vi "Lab6_DPSK2.vi"() -> ()   [LabVIEW 2019]
uses:
  <vilib>/addons/Modulation/Analog/support/mod_Set Error Source.vi
  <vilib>/addons/Modulation/Digital/Support/Common/Validators/mod_AWGN Validate.vi
  <vilib>/addons/Modulation/Digital/Impairments/subVIs/mod_createSeeds.vi
  <vilib>/addons/Modulation/Digital/Support/Common/Validators/mod_Validate Samples Per Symbol.vi
  <vilib>/addons/Modulation/Analog/support/Validators/mod_Validate Complex Waveform.vi
  <vilib>/addons/Modulation/Analog/support/Validators/mod_WFErrorHandler.vi
  <vilib>/addons/Modulation/Digital/Support/Common/Validators/mod_Generate Filter Coefficients Validate.vi
  <vilib>/addons/Modulation/Digital/General/subVIs/mod_Generate Filter Coefficients.vi
  <vilib>/addons/Modulation/Digital/General/MT Generate PSK System Parameters(M).vi
  <vilib>/addons/Modulation/Digital/General/MT Generate PSK Synchronization Parameters (bit array).vi
  <vilib>/addons/Modulation/Digital/General/subVIs/mod_Generate Bits PN Sequence.vi
  <vilib>/Analysis/1siggen.llb/Gaussian White Noise (obs 90).vi
  <vilib>/addons/Modulation/Analog/MT Upconvert Baseband (Real).vi
  <vilib>/addons/Modulation/Digital/Demodulation/MT Calculate BER After Trigger (PN Sequence).vi
  <vilib>/addons/Modulation/Digital/General/MT Format Eye Diagram (complex).vi
  <vilib>/express/express analysis/Spectral/Block/exnSpectralBlock spectral measurements RMS poly.vi
  <vilib>/express/express analysis/Spectral/Block/exnSpectralBlock spectral measurements RMS WFM.vi
  <vilib>/express/express analysis/Spectral/XNode/ExpressSpectralMeasurementsBlockNode.xnode
  <vilib>/addons/Modulation/niDMT.lvlib
  <vilib>/addons/Modulation/niAMT.lvlib
panel:
  in  "Tab Control 2":T1(tab)
  out "bassband wfm1":cluster{"t0":dbl, "dt":dbl, "Y":dbl[]}(graph)
  out "bassband wfm2":cluster{"t0":dbl, "dt":dbl, "Y":dbl[]}(graph)
  out "passband wfm":waveform(dbl)(graph)
  out "Spectral":cluster{"f0":dbl, "df":dbl, "magnitude":dbl[]}(graph)
  in  "Tab Control":enum32{" Constellation", "Eye Diagram"}(tab)
  out "Constellation":T2(graph)
  out "Eye Diagram":cluster{"t0":dbl, "dt":dbl, "Y":dbl[]}[](graph)
  in  "carrier frequency (Hz)":dbl min=-0.5 max=0.5 format="%.0p"
  in  "PSK type":u16(ring) items=["normal", "shifted", "offset"]
  out "Transmitted bitstream":i8[](array[numeric])
  out "Receive bit stream":i8[](array[numeric])
  in  "Eb/N0 (10 dB)":dbl(knob)=10.0 scale=0.0..60.0
  in  "symbol rate (Hz)":dbl=1.0 format="%.0p"
  in  "M-PSK(4)":i32(ring) items=["2"=2, "4"=4, "8"=8, "16"=16]
  in  "stop":bool
  in  "pulse shaping filter":u16(ring) items=["none", "Raised Cosine", "Root Raised Cos", "Gaussian"]
  # "DPSK and Offset-PSK"
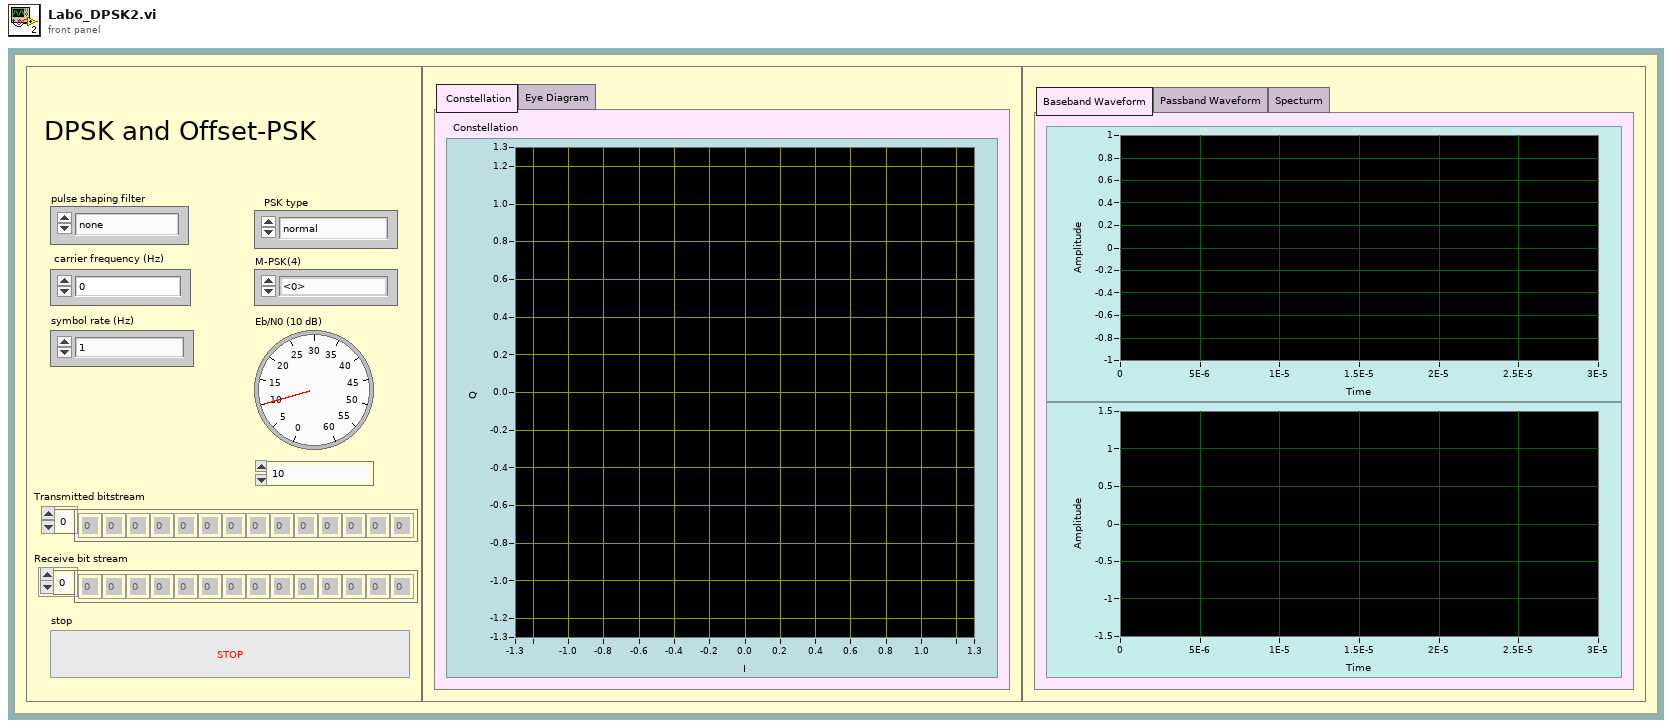
[diagram p1: front panel]
types:
  T1 = enum32{"Baseband Waveform", "Passband Waveform", "Specturm"}
  T2 = cluster{"Decimated Array":dbl[], "Decimated Array":dbl[]}[]
  T3 = enum16{"FSK", "PSK", "QAM", "MSK", "PAM", "ASK", "CPM"}
  T4 = cluster{"averaging mode":u16, "weighting mode":u16, "number of averages":u32}
  T5 = cluster{"dB On (F)":bool, "unwrap phase (F)":bool, "convert to degree (F)":bool}
  T6 = cluster{"samples per symbol (16)":i32, "symbol map":cdb[], "differential PSK":enum16{"disable", "enable"}, "PSK type":u16}
  T7 = cluster{"expected sync location (symbols)":i32, "sync sequence":cdb[], "sync location uncertainty (symbols)":i32, "sync indent (symbols)":i32}
  T8 = typedef "niAMT.lvlib/Complex Data Waveform.ctl" = cluster{"t0":dbl, "dt":dbl, "Y":cdb[]}
  T9 = cluster{"constellation":dbl[], "oversampled data":dbl[]}[]
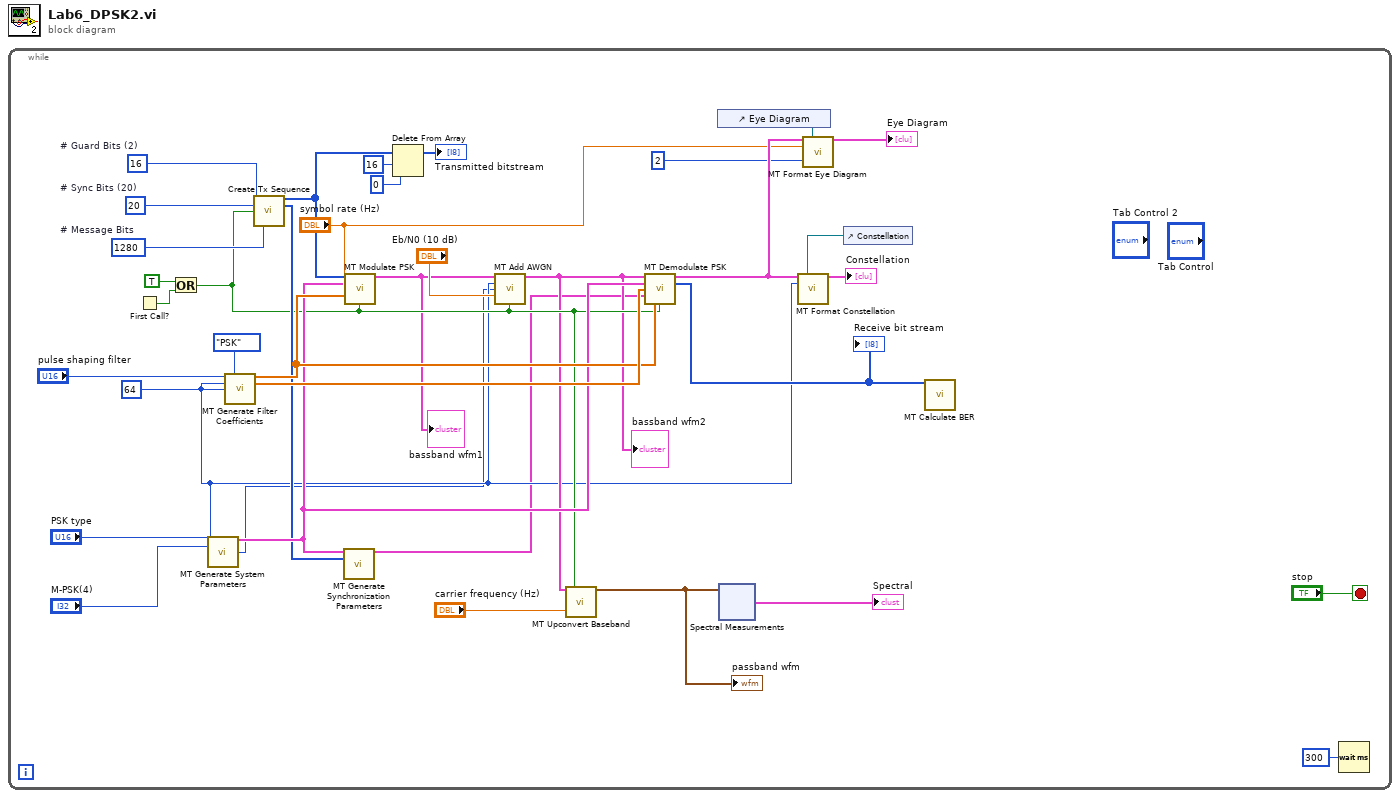
[diagram p0: block diagram]
diagram:
  n1 = while {
    stop <- "stop" stop-if-true
    w4 = 64 ("pulse shaping samples per symbol (16)")
    w12 = 16  # # Guard Bits (2)
    w13 = 1280  # # Message Bits
    w14 = 20  # # Sync Bits (20)
    n2 = First Call?() -> (First Call?: T/F=w10:bool)
    n3 = Or(x=TRUE, y=w10) -> (x .or. y?=w8:bool)
    n4 = call-poly <vilib>:"MT Generate System Parameters.vi"("samples per symbol (16)"=w4, "PSK type"="PSK type", "M-PSK (4)"="M-PSK(4)") -> ("PSK system parameters"=w19:T6, "bits per symbol"=w3:i32)  [unwired: 10 in, 1 out]
    n5 = call <vilib>:"MT Generate Filter Coefficients.vi"("pulse shaping filter (none)"="pulse shaping filter", "modulation type"=T3."PSK", "pulse shaping samples per symbol (16)"=w4, "matched samples per symbol (16)"=w4) -> ("pulse shaping filter coefficients"=w20:dbl[], "matched filter coefficients"=w21:dbl[])  [unwired: 9 in, 1 out]
    n6 = call "Create Tx Sequence.vi"("# Guard Bits (2)"=w12, "# Sync Bits (20)"=w14, "Reset? (T)"=w8, "# Message Bits"=w13) -> ("Output Bit Stream"=w27:i8[], "Last Sync Pattern"=w16:i8[])  [unwired: 8 in, 2 out]
    n7 = call-poly <vilib>:"MT Generate Synchronization Parameters.vi"("PSK system parameters"=w19, "sync bits"=w16) -> ("PSK synchronization parameters"=w2:T7)  [unwired: 12 in, 1 out]
    n8 = call <vilib>:"MT Modulate PSK.vi"("input bit stream"=w27, "PSK system parameters"=w19, "symbol rate (Hz)"="symbol rate (Hz)", "pulse shaping filter coefficients"=w20, "reset? (T)"=w8) -> ("output complex waveform"=w6:T8)  [unwired: 8 in, 2 out]
    "bassband wfm1" <- w6
    n9 = Delete From Array(array=w27, length=16, index=0) -> (array with subset deleted=→"Transmitted bitstream":i8[])  [unwired: 1 out]
    n10 = call <vilib>:"MT Add AWGN.vi"("input complex waveform"=w6, "samples per symbol (16)"=w4, "bits per symbol (1)"=w3, "Eb/N0 (10 dB)"="Eb/N0 (10 dB)", "reset? (T)"=w8) -> ("output complex waveform"=w5:T8)  [unwired: 8 in, 2 out]
    "bassband wfm2" <- w5
    n11 = call-poly <vilib>:"MT Upconvert Baseband.vi"("baseband waveform (complex)"=w5, "reset? (F)"=w8, "carrier frequency (Hz)"="carrier frequency (Hz)") -> ("passband waveform"=w7:waveform(dbl))  [unwired: 11 in, 1 out]
    "passband wfm" <- w7
    n12 = call <vilib>:"MT Demodulate PSK.vi"("input complex waveform"=w5, "PSK system parameters"=w19, "matched filter coefficients"=w21, "synchronization parameters"=w2, "pulse shaping filter coefficients"=w20, "reset? (T)"=w8) -> ("recovered complex waveform"=w25:T8, "output bit stream"=w18:i8[])  [unwired: 5 in, 3 out]
    "Receive bit stream" <- w18
    n13 = control-ref of="Eye Diagram"() -> (w33:refnum<vi>)
    n14 = xnode "Spectral Measurements"("Signals"=w7) -> ("Measurement Output"=→"Spectral":cluster{"f0":dbl, "df":dbl, "magnitude":dbl[]})  [unwired: 1 in, 2 out]
    n15 = call-poly <vilib>:"MT Format Eye Diagram.vi"("waveform"=w25, "eye diagram reference"=w33, "symbol rate (Hz)"="symbol rate (Hz)", "eye length"=2) -> ("eye diagram"=→"Eye Diagram":cluster{"t0":dbl, "dt":dbl, "Y":dbl[]}[])  [unwired: 3 in, 8 out]
    n16 = control-ref of="Constellation"() -> (w36:refnum<vi>)
    n17 = call <vilib>:"MT Format Constellation.vi"("waveform"=w25, "constellation reference"=w36, "samples per symbol"=w4) -> ("constellation graph"=→"Constellation":T9)  [unwired: 2 in, 10 out]
    n18 = call-poly <vilib>:"MT Calculate BER.vi"("input bit stream"=w18) -> ()  [unwired: 10 in, 5 out]
    n19 = Wait (ms)(milliseconds to wait=u32 300) -> ()  [unwired: 1 out]
  }
